vi "Overlay LineOut from ROI.vi"(0 "Image In":T4, 1 "ROI":T2, 2 "Font, Size & Style":T1={"Desired Font (Application)"=enum."Application Font", "[User-specified Font]"={"Font Name"="", "Size"=12, "Strikeout?"=FALSE, "Italic?"=FALSE, "Underline?"=FALSE, "Outline?"=FALSE, "Shadow?"=FALSE, "Bold?"=FALSE, "Rotation Angle"=0.0}, "Horizontal Alignment"=0, "Vertical Alignment"=0} {"Vertical Alignment" items=["Bottom", "Top", "Baseline"]; "Horizontal Alignment" items=["Left", "Center", "Right"]; "[User-specified Font]"."Rotation Angle" format="%.2f"}, 3 "Calbration":dbl[unit]=1e-06, 4 "Group":string, 5 "error in":errorcluster) -> (6 "Image Out":T4, 7 "FWHM":dbl[](array[numeric]), 8 "error out":errorcluster)   [LabVIEW 2020, in "POLARIS Vision utility.lvlib"]
doc: "Filters ROI countours of line type and shows their lineotus like a trend with arbitary units. If slope of the line is les 45° trend appears at bottom border otherwise at the left border. \n\nthanks for idee and first implementation to Sebastian Keppler, FSU-IOQ\n\nauthor: Alexander Kessler, Helmholtz-Institut-Jena \nmaintainer: Alexander Kessler: alexander.kessler@uni-jena.de\n\n\n\nLicense Agreement for this software:\n\nCopyright (C)\nHelmholtz-Institut-Jena\nFröbelstieg 3\n07743 Jena\nGermany\n\nThis program is free software; you can redistribute it and/or modify it under the terms of the GNU General Public License as published by the Free Software Foundation; either version 2 of the license, or (at your option) any later version.\n\nThis program is distributed in the hope that it will be useful, but WITHOUT ANY WARRANTY; without even the implied warranty of MERCHANTABILITY or FITNESS FOR A PARTICULAR PURPOSE. See the GNU General License for more details (http://www.gnu.org)."
uses:
  POLARIS Vision utility.lvlib
  <vilib>/vision/Image Controls.llb/IMAQ Image.ctl
panel:
  out "Waveform Graph":T3(graph)
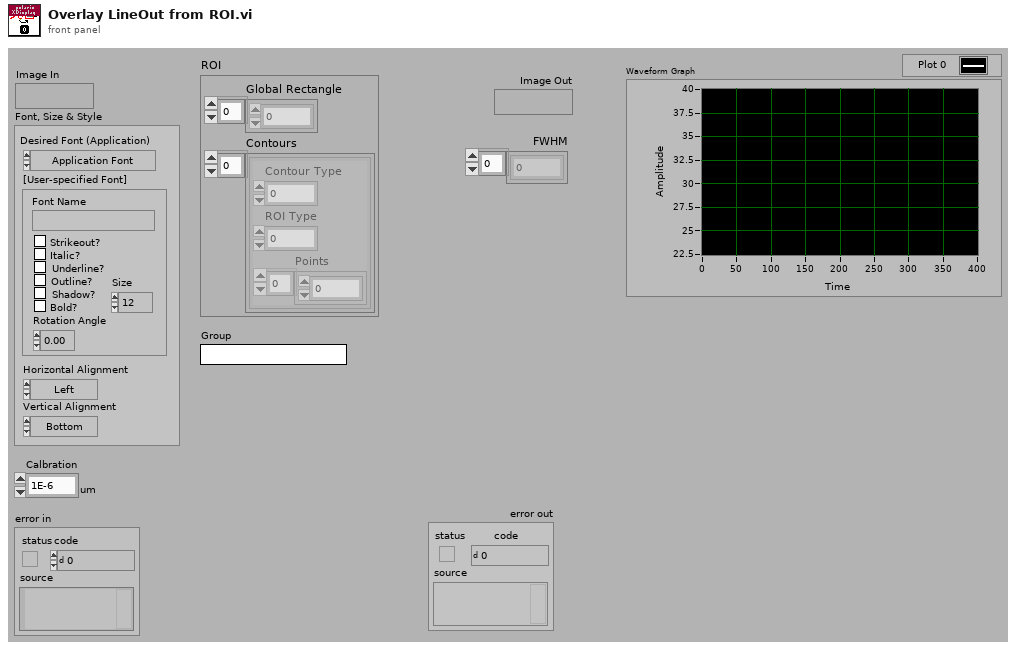
[diagram p1: front panel]
types:
  T1 = cluster{"Desired Font (Application)":enum16{"User-specified Font", "Application Font", "System Font", "Dialog Font"}, "[User-specified Font]":cluster{"Font Name":string, "Size":i16, "Strikeout?":bool, "Italic?":bool, "Underline?":bool, "Outline?":bool, "Shadow?":bool, "Bold?":bool, "Rotation Angle":dbl}, "Horizontal Alignment":i16, "Vertical Alignment":i16}
  T2 = cluster{"Global Rectangle":i32[], "Contours":cluster{"Contour Type":u32, "ROI Type":u32, "Points":i32[]}[]}
  T3 = cluster{"x0":sgl, "dx":sgl, "Pixels Line":sgl[]}[]
  T4 = typedef "IMAQ Image.ctl" = refnum<image>
  T5 = cluster{"Contour Type":u32, "ROI Type":u32, "Points":i32[]}[]
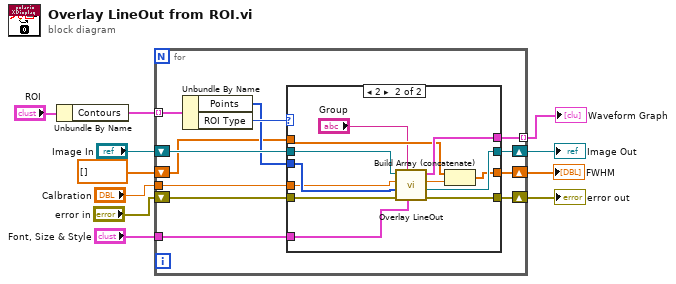
[diagram p0: block diagram]
diagram:
  n1 = Unbundle By Name("ROI") -> ("Contours"=w11:T5)
  n2 = for {
    tunnel: w11 -> [w23] mode=indexing
    tunnel: [w19] -> w10 mode=indexing
    shift-right: [w18] -> w7
    shift-left: "Image In" -> [w21]
    shift-right: [w16] -> w6
    shift-left: dbl[] [] -> [w17]
    shift-right: [w14] -> w3
    shift-left: "error in" -> [w15]
    tunnel: "Calbration" -> [w13]
    tunnel: "Font, Size & Style" -> [w12]
    n3 = Unbundle By Name(w23) -> ("Points"=w20:i32[], "ROI Type"=w22:u32)
    n4 = case shown="2" w22 {
      tunnel: w21 -> [w26 w38]
      tunnel: w20 -> [_ w36]
      tunnel: [_ w35] -> w19
      tunnel: [w26 w37] -> w18
      tunnel: w17 -> [w25 w34]
      tunnel: [w25 w33] -> w16
      tunnel: w15 -> [w24 w31]
      tunnel: [w24 w30] -> w14
      tunnel: w13 -> [_ w28]
      tunnel: w12 -> [_ w27]
      frame 0, Default {
      }
      frame 2 {
        n5 = call "Overlay LineOut.vi"("Font, Size & Style"=w27, "Group"="Group", "error in"=w31, "LineCoord"=w36, "Calibration"=w28, "Image In"=w38) -> ("error out"=w30:errorcluster, "Image Out"=w37:T4, "FWHM"=w32:dbl, "Line Graph"=w35:cluster{"x0":sgl, "dx":sgl, "Pixels Line":sgl[]})  [unwired: 2 in]
        n6 = Build Array (concatenate)(w34, w32) -> (w33:dbl[])
      }
    }
  }
  "Image Out" <- w7
  "Waveform Graph" <- w10
  "FWHM" <- w6
  "error out" <- w3
